vi "sendDigitalOutputs.vi"(8 "error in (no error)":errorcluster, 11 "ILC in":refnum<class "ILC.lvclass">) -> (0 "error out":errorcluster, 3 "ILC out":refnum<class "ILC.lvclass">)   [LabVIEW 2015, in "ILCCommon.lvlib" / "ILC.lvclass"]
uses:
  <userlib>/Common/ILC/ILC/ILC.lvclass
  <userlib>/Common/ILC/ILC/ILC.lvclass/ILC.ctl
  <userlib>/Common/SerialProtocols/SerialCommunicator/SerialCommunicator.lvclass
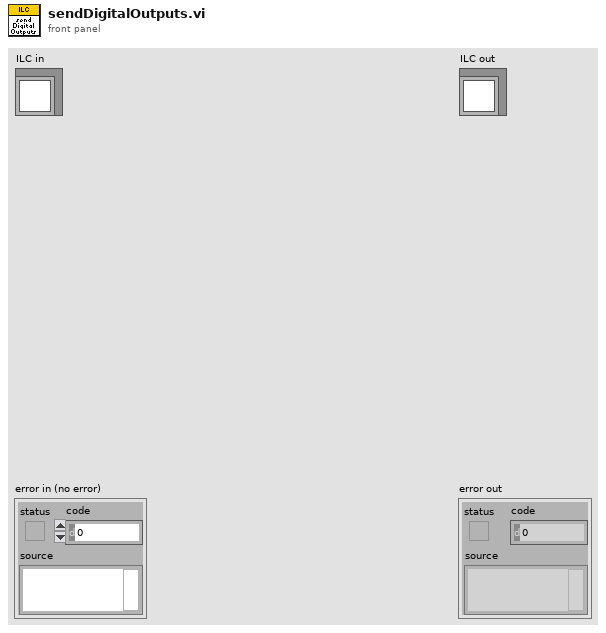
[diagram p1: front panel]
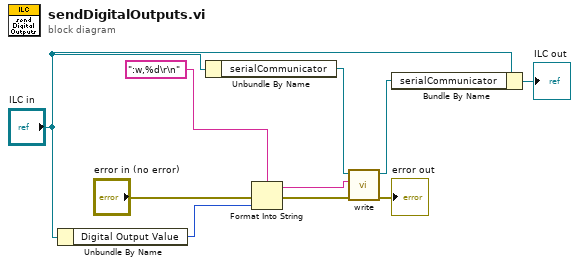
[diagram p0: block diagram]
diagram:
  n1 = Unbundle By Name("ILC in") -> ("Digital Output Value"=w1:i32)
  n2 = Unbundle By Name("ILC in") -> ("serialCommunicator"=w8:refnum<class "SerialCommunicator.lvclass">)
  n3 = Format Into String(format string=":w,%d\r\n", error in="error in (no error)", w1) -> (resulting string=w10:string, error out=w5:errorcluster)  [unwired: 1 in]
  n4 = call-dynamic "write.vi"("error in (no error)"=w5, "writeString"=w10, "SerialCommunicator in"=w8) -> ("error out"=→"error out":errorcluster, "SerialCommunicator out"=w3:refnum<class "SerialCommunicator.lvclass">)  [unwired: 7 in]
  n5 = Bundle By Name(cluster="ILC in", "serialCommunicator"=w3) -> (→"ILC out":refnum<class "ILC.lvclass">)
